vi "Main.vi"() -> ()   [LabVIEW 2019]
doc: "This template is for the Queued Message Handler design pattern.\n\nThe Event Handling Loop generates messages based on user interface actions.\n\nThe Message Handling Loop processes messages generated by the Event Handling Loop, or by other messages. The messages are string values, so new messages can be added easily to the Message Cases case structure in the Message Handling Loop. Each message cluster can also provide an optional value for Message Data, which is a variant that can be converted to whatever message-specific data is required."
uses:
  controls/UI Data.ctl
  support/Message Queue/Enqueue Message (Single).vi
  <vilib>/Utility/error.llb/Error Cluster From Error Code.vi
  <vilib>/ErrorRing/Error Ring.xnode
  support/Message Queue/Message Queue.lvlib
  support/User Event - Stop/User Events.lvlib
panel:
  out "Volts":dbl(knob) scale=0.0..10.0
  out "Display <Replace Me>":string
  in  "Do Something Else <Replace Me>":bool
  in  "Do Something <Replace Me>":bool
  in  "Exit":bool
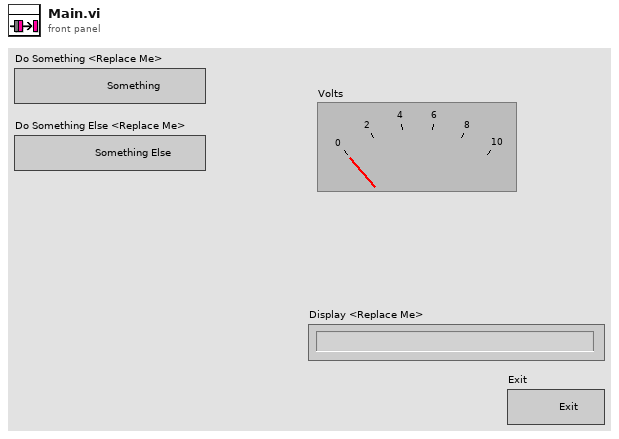
[diagram p1: front panel]
types:
  T1 = typedef "UI Data.ctl" = cluster{"Boolean <Replace Me>":bool, "String <Replace Me>":string, "Numeric <Replace Me>":dbl, "Do Something Ref":refnum<vi>, "Do Something Else Ref":refnum<vi>, "Data Display Ref":refnum<vi>, "Exit Button Ref":refnum<vi>}
  T2 = typedef "User Events.lvlib/User Events Typedef.ctl" = cluster{"Stop Event Interno":refnum<user-event>, "Volts":refnum<user-event>, "QMH Stop":refnum<user-event>, "Stop Event Externo":refnum<user-event>}
  T3 = typedef "Message Queue.lvlib/All Message Queues.ctl" = cluster{"UI":refnum<queue>}
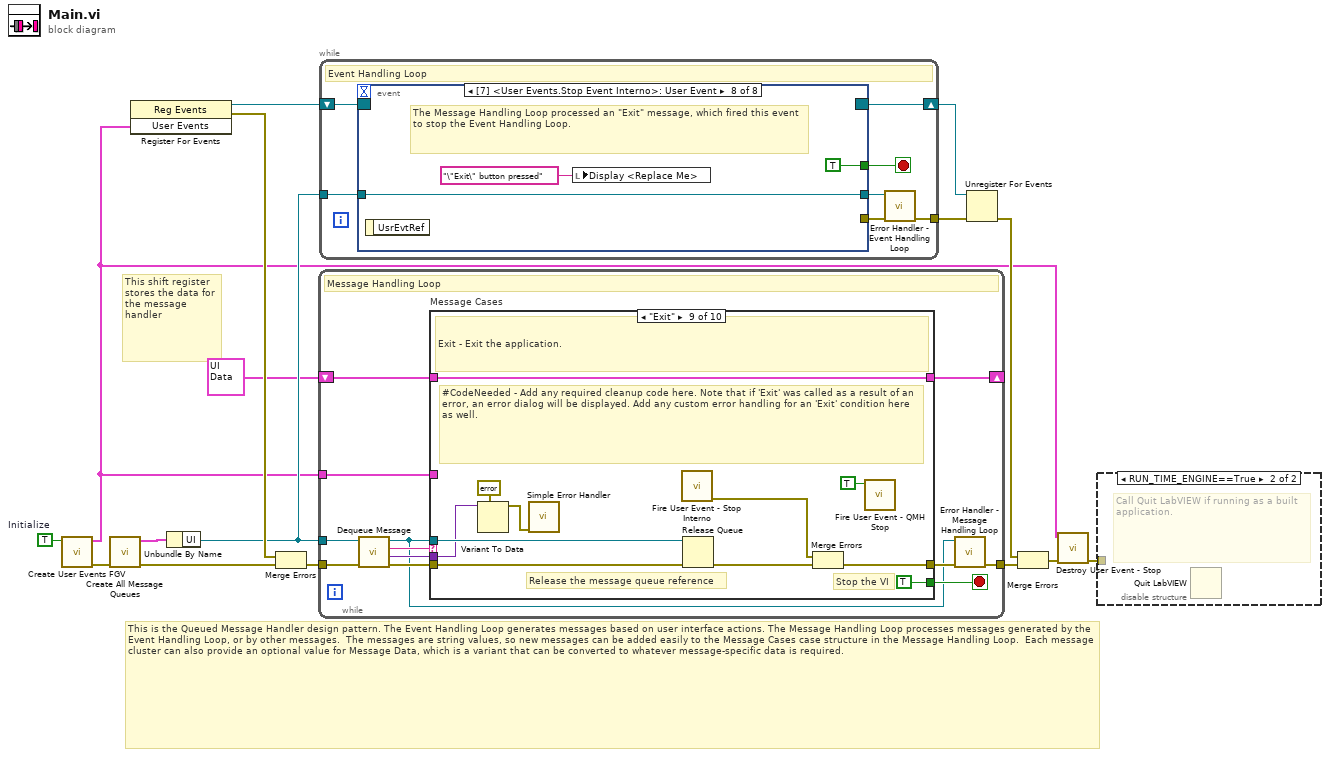
[diagram p0: block diagram]
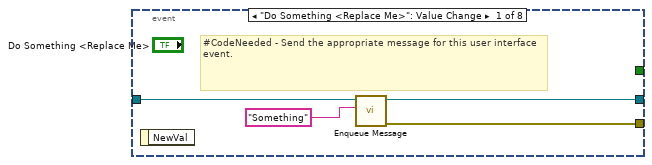
[diagram p3: hidden frame]
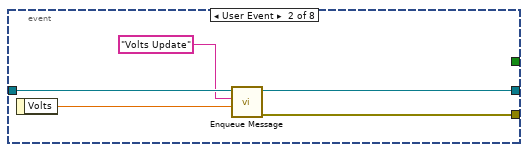
[diagram p4: hidden frame]
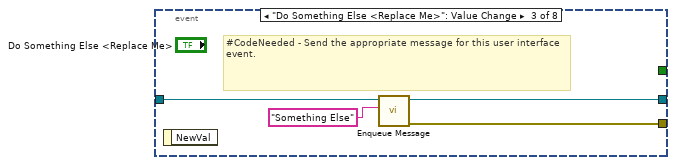
[diagram p5: hidden frame]
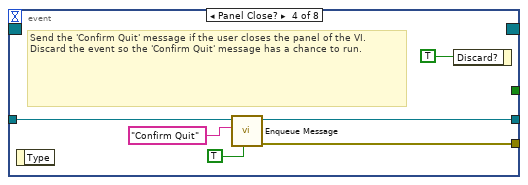
[diagram p6: hidden frame]
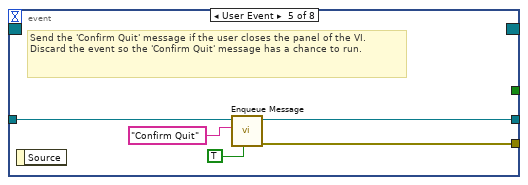
[diagram p7: hidden frame]
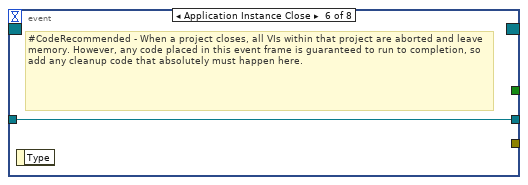
[diagram p8: hidden frame]
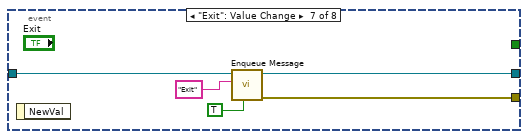
[diagram p9: hidden frame]
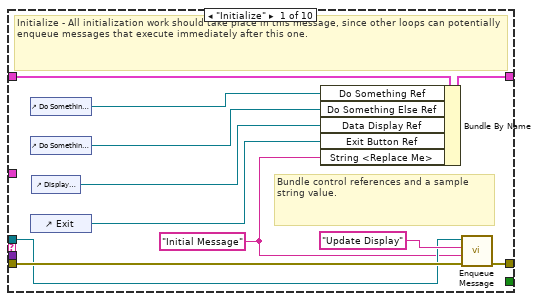
[diagram p10: hidden frame]
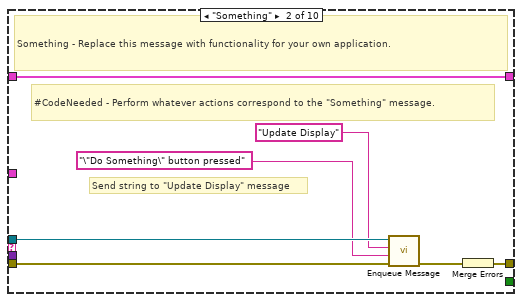
[diagram p11: hidden frame]
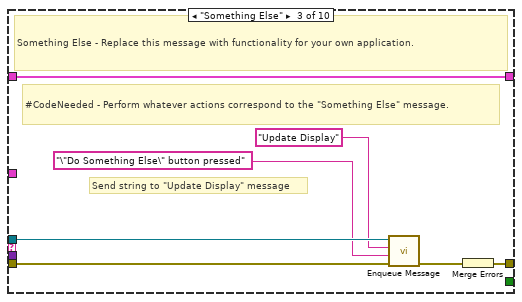
[diagram p12: hidden frame]
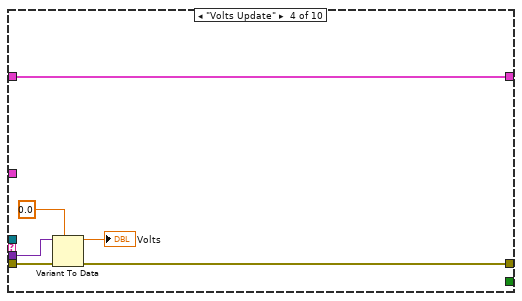
[diagram p13: hidden frame]
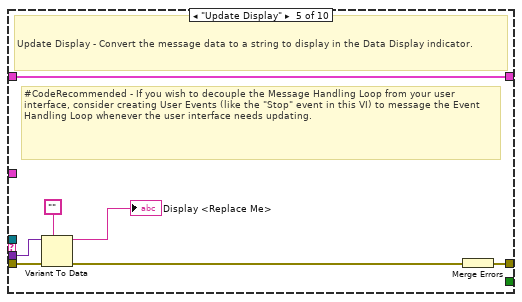
[diagram p14: hidden frame]
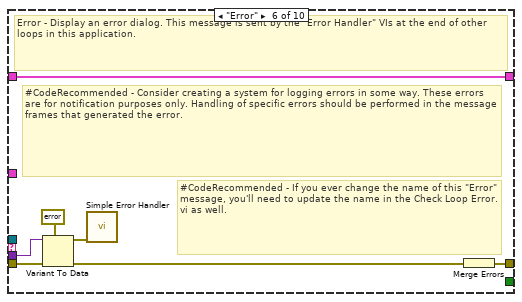
[diagram p15: hidden frame]
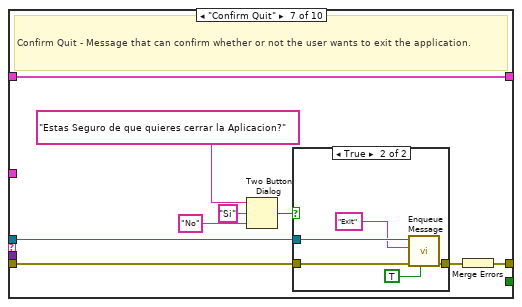
[diagram p16: hidden frame]
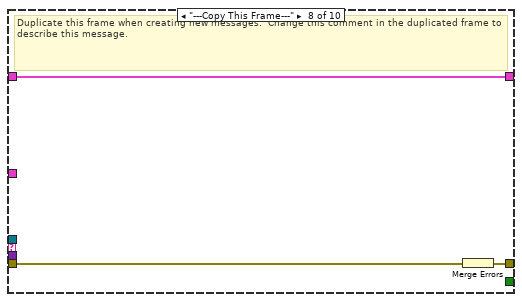
[diagram p18: hidden frame]
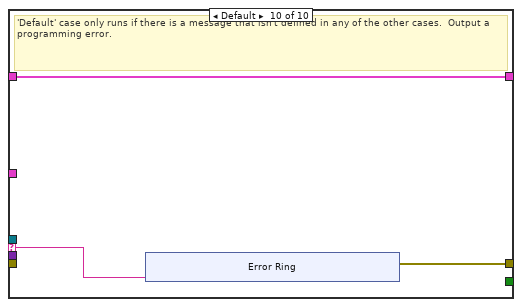
[diagram p19: hidden frame]
diagram:
  w1 = TRUE  # Initialize
  # "This is the Queued Message Handler design pattern. The Event Handling Loop generates messages based on user interface actions. The Message Handling Loop processes messages generated by the Event Handling Loop, or by other messages.  The messages are string values, so new messages can be added easily to the Message Cases case structure in the Message Handling Loop.  Each message cluster can also provide an optional value for Message Data, which is a variant that can be converted to whatever message-specific data is required."
  # "This shift register stores the data for the message handler"
  n1 = call "Create User Events FGV.vi"("Initialize"=w1) -> ("error out"=w14:errorcluster, "User Events"=w2:T2)  [unwired: 9 in]
  n2 = call "Create All Message Queues.vi"("error in (no error)"=w14) -> ("error out"=w16:errorcluster, "Message Queues out"=w7:T3)  [unwired: 9 in]
  n3 = register-events(w2) -> (reference out=w3:refnum<event-registration>, error out=w8:errorcluster)  [unwired: 2 in]
  n4 = Unbundle By Name(w7) -> ("UI"=w6:refnum<queue>)
  n5 = Merge Errors(w8, w16) -> (w9:errorcluster)
  n6 = while {
    tunnel: w6 -> [w18]
    shift-right: [w23] -> _
    shift-left: T1 {"Boolean <Replace Me>"=FALSE, "String <Replace Me>"="", "Numeric <Replace Me>"=0.0, "Do Something Ref"=refnum, "Do Something Else Ref"=refnum, "Data Display Ref"=refnum, "Exit Button Ref"=refnum} ("Data Cluster") -> [w24]
    tunnel: w2 -> [w21]
    tunnel: w9 -> [w28]
    tunnel: [w26] -> w15
    stop <- w22 stop-if-true
    # "Message Handling Loop"
    n7 = call "Dequeue Message.vi"("error in (no error)"=w28, "Message Queue"=w18) -> ("error out"=w27:errorcluster, "Message Data"=w19:variant, "Message"=w20:string, "dup Message Queue"=w17:refnum<queue>)  [unwired: 6 in]
    n8 = case "Message Cases" shown="\"Exit\"" w20 {
      selector: w20 -> [_ _ _ _ _ _ _ _ _ w103]
      tunnel: w17 -> [w30 w42 w49 _ _ _ w78 _ w96 _]
      tunnel: w27 -> [w38 w45 w52 w59 w65 w73 w82 w91 w99 _]
      tunnel: [w39 w46 w53 w58 w66 w69 w81 w90 w101 w105] -> w25
      tunnel: w24 -> [w37 w43 w50 w57 w63 w68 w79 w89 w95 w104]
      tunnel: [w36 w43 w50 w57 w63 w68 w79 w89 w95 w104] -> w23
      tunnel: [_ _ _ _ _ _ _ _ TRUE _] -> w22
      tunnel: w19 -> [_ _ _ w56 w62 w67 _ _ w93 _]
      tunnel: w21 -> [_ _ _ _ _ _ _ _ _ _]
      frame "Initialize" {
        w29 = "Initial Message" ("Initial Message")
        # "Bundle control references and a sample string value."
        # "Initialize - All initialization work should take place in this message, since other loops can potentially enqueue messages that execute immediately after this one."
        n9 = control-ref of="Do Something <Replace Me>"() -> (w35:refnum<vi>)
        n10 = control-ref of="Do Something Else <Replace Me>"() -> (w34:refnum<vi>)
        n11 = control-ref of="Exit"() -> (w32:refnum<vi>)
        n12 = control-ref of="Display <Replace Me>"() -> (w33:refnum<vi>)
        n13 = Bundle By Name(cluster=w37, "Do Something Ref"=w35, "Do Something Else Ref"=w34, "Data Display Ref"=w33, "Exit Button Ref"=w32, "String <Replace Me>"=w29) -> (w36:T1)
        n14 = call-poly "Enqueue Message.vi"("error in (no error)"=w38, "Message Data"=w29, "Message"="Update Display", "Message Queue"=w30) -> ("error out"=w39:errorcluster)  [unwired: 6 in, 1 out]
      }
      frame "Something" {
        # "Send string to \"Update Display\" message"
        # "#CodeNeeded - Perform whatever actions correspond to the \"Something\" message."
        # "Something - Replace this message with functionality for your own application."
        n15 = call-poly "Enqueue Message.vi"("error in (no error)"=w45, "Message Data"="\"Do Something\" button pressed" ("\"Do Something\" button pressed"), "Message"="Update Display", "Message Queue"=w42) -> ("error out"=w44:errorcluster)  [unwired: 6 in, 1 out]
        n16 = Merge Errors(w44) -> (w46:errorcluster)
      }
      frame "Something Else" {
        # "Send string to \"Update Display\" message"
        # "#CodeNeeded - Perform whatever actions correspond to the \"Something Else\" message."
        # "Something Else - Replace this message with functionality for your own application."
        n17 = call-poly "Enqueue Message.vi"("error in (no error)"=w52, "Message Data"="\"Do Something Else\" button pressed" ("\"Do Something Else\" button pressed"), "Message"="Update Display", "Message Queue"=w49) -> ("error out"=w51:errorcluster)  [unwired: 6 in, 1 out]
        n18 = Merge Errors(w51) -> (w53:errorcluster)
      }
      frame "Volts Update" {
        n19 = Variant To Data(error in=w59, type=0.0, Variant=w56) -> (data=→"Volts":dbl, error out=w58:errorcluster)
      }
      frame "Update Display" {
        # "#CodeRecommended - If you wish to decouple the Message Handling Loop from your user interface, consider creating User Events (like the \"Stop\" event in this VI) to message the Event Handling Loop whenever the user interface needs updating."
        # "Update Display - Convert the message data to a string to display in the Data Display indicator."
        n20 = Variant To Data(error in=w65, type="", Variant=w62) -> (data=→"Display <Replace Me>":string, error out=w64:errorcluster)
        n21 = Merge Errors(w64) -> (w66:errorcluster)
      }
      frame "Error" {
        # "#CodeRecommended - If you ever change the name of this \"Error\" message, you'll need to update the name in the Check Loop Error.vi as well."
        # "#CodeRecommended - Consider creating a system for logging errors in some way. These errors are for notification purposes only. Handling of specific errors should be performed in the message frames that generated the error."
        # "Error - Display an error dialog. This message is sent by the \"Error Handler\" VIs at the end of other loops in this application."
        n22 = Variant To Data(error in=w73, type=errorcluster {"status"=FALSE, "code"=0, "source"=""} ("error constant"), Variant=w67) -> (data=w71:errorcluster, error out=w70:errorcluster)
        n23 = call <vilib>:"Simple Error Handler.vi"("error in (no error)"=w71) -> ()  [unwired: 4 in, 5 out]
        n24 = Merge Errors(w70) -> (w69:errorcluster)
      }
      frame "Confirm Quit" {
        # "Confirm Quit - Message that can confirm whether or not the user wants to exit the application."
        n25 = Two Button Dialog(message="Estas Seguro de que quieres cerrar la Aplicacion?", 1:"No" ("T button name (\"OK\")"), 2:"Si" ("T button name (\"OK\")")) -> (T button?=w77:bool)
        n26 = case shown="True" w77 {
          tunnel: w82 -> [w83 w88]
          tunnel: [w83 w87] -> w80
          tunnel: w78 -> [_ w86]
          frame False {
          }
          frame True {
            n27 = call-poly "Enqueue Message.vi"("Priority Message? (F)"=TRUE, "error in (no error)"=w88, "Message"="Exit", "Message Queue"=w86) -> ("error out"=w87:errorcluster)  [unwired: 6 in, 1 out]
          }
        }
        n28 = Merge Errors(w80) -> (w81:errorcluster)
      }
      frame "---Copy This Frame---" {
        # "Duplicate this frame when creating new messages.  Change this comment in the duplicated frame to describe this message."
        n29 = Merge Errors(w91) -> (w90:errorcluster)
      }
      frame "Exit" {
        # "Stop the VI"
        # "Release the message queue reference"
        # "#CodeNeeded - Add any required cleanup code here. Note that if 'Exit' was called as a result of an error, an error dialog will be displayed. Add any custom error handling for an 'Exit' condition here as well."
        # "Exit - Exit the application."
        n30 = Variant To Data(type=errorcluster {"status"=FALSE, "code"=0, "source"=""} ("error constant"), Variant=w93) -> (data=w97:errorcluster)  [unwired: 1 in, 1 out]
        n31 = call <vilib>:"Simple Error Handler.vi"("error in (no error)"=w97) -> ()  [unwired: 4 in, 5 out]
        n32 = call "Fire User Event - Stop Interno.vi"() -> ("error out"=w100:errorcluster)  [unwired: 11 in]
        n33 = Release Queue(queue=w96, error in (no error)=w99) -> (error out=w102:errorcluster)  [unwired: 1 in, 2 out]
        n34 = Merge Errors(w100, w102) -> (w101:errorcluster)
        n35 = call "Fire User Event - QMH Stop.vi"("QMH Stop"=TRUE) -> ()  [unwired: 10 in, 1 out]
      }
      frame Default {
        # "'Default' case only runs if there is a message that isn't defined in any of the other cases.  Output a programming error."
        n36 = xnode "Error Ring"("parameter 0"=w103) -> ("error out"=w105:errorcluster)
      }
    }
    n37 = call "Error Handler - Message Handling Loop.vi"("error in (no error)"=w25, "Message Queue"=w17) -> ("dup error in"=w26:errorcluster)  [unwired: 8 in, 1 out]
  }
  n38 = while {
    tunnel: w6 -> [w117]
    shift-right: [w115] -> w5
    shift-left: w3 -> [w116]
    tunnel: [w118] -> w10
    stop <- w114 stop-if-true
    # "Event Handling Loop"
    n39 = event shown="[7] <User Events.Stop Event Interno>: User Event" {
      selector: w116 -> [_ _ _ _ _ _ _ _]
      dyn-events: [_ _ _ _ _ _ _ _] -> w115
      timeout: _ -> [_ _ _ _ _ _ _ _]
      tunnel: [_ _ _ _ _ _ _ TRUE ("Discard?")] -> w114
      tunnel: w117 -> [w122 w127 w131 w136 w142 w144 w148 w152]
      tunnel: [w123 w128 w132 w138 w143 _ w149 _] -> w119
      tunnel: [w121 w126 w130 w135 w141 w144 w147 w152] -> w113
      event "Do Something <Replace Me>": Value Change {
        # "#CodeNeeded - Send the appropriate message for this user interface event."
        n40 = event-data() -> ()  [unwired: 1 in, 1 out]
        n41 = call-poly "Enqueue Message.vi"("Message"="Something", "Message Queue"=w122) -> ("error out"=w123:errorcluster, "dup Message Queue"=w121:refnum<queue>)  [unwired: 8 in]
      }
      event User Event {
        n42 = event-data() -> ("Volts"=w124:dbl)  [unwired: 1 in]
        n43 = call-poly "Enqueue Message.vi"("Message Data"=w124, "Message"="Volts Update", "Message Queue"=w127) -> ("error out"=w128:errorcluster, "dup Message Queue"=w126:refnum<queue>)  [unwired: 7 in]
      }
      event "Do Something Else <Replace Me>": Value Change {
        # "#CodeNeeded - Send the appropriate message for this user interface event."
        n44 = event-data() -> ()  [unwired: 1 in, 1 out]
        n45 = call-poly "Enqueue Message.vi"("Message"="Something Else", "Message Queue"=w131) -> ("error out"=w132:errorcluster, "dup Message Queue"=w130:refnum<queue>)  [unwired: 8 in]
      }
      event Panel Close? {
        # "Send the 'Confirm Quit' message if the user closes the panel of the VI. Discard the event so the 'Confirm Quit' message has a chance to run."
        n46 = event-data() -> ()  [unwired: 1 in, 1 out]
        n47 = call-poly "Enqueue Message.vi"("Priority Message? (F)"=TRUE, "Message"="Confirm Quit", "Message Queue"=w136) -> ("error out"=w138:errorcluster, "dup Message Queue"=w135:refnum<queue>)  [unwired: 7 in]
        n48 = event-data("Discard?"=TRUE) -> ()  [unwired: 1 in, 1 out]
      }
      event User Event {
        # "Send the 'Confirm Quit' message if the user closes the panel of the VI. Discard the event so the 'Confirm Quit' message has a chance to run."
        n49 = event-data() -> ()  [unwired: 1 in, 1 out]
        n50 = call-poly "Enqueue Message.vi"("Priority Message? (F)"=TRUE, "Message"="Confirm Quit", "Message Queue"=w142) -> ("error out"=w143:errorcluster, "dup Message Queue"=w141:refnum<queue>)  [unwired: 7 in]
      }
      event Application Instance Close {
        # "#CodeRecommended - When a project closes, all VIs within that project are aborted and leave memory. However, any code placed in this event frame is guaranteed to run to completion, so add any cleanup code that absolutely must happen here."
        n51 = event-data() -> ()  [unwired: 1 in, 1 out]
      }
      event "Exit": Value Change {
        n52 = event-data() -> ()  [unwired: 1 in, 1 out]
        n53 = call-poly "Enqueue Message.vi"("Priority Message? (F)"=TRUE, "Message"="Exit", "Message Queue"=w148) -> ("error out"=w149:errorcluster, "dup Message Queue"=w147:refnum<queue>)  [unwired: 7 in]
      }
      event User Event {
        # "The Message Handling Loop processed an \"Exit\" message, which fired this event to stop the Event Handling Loop."
        n54 = event-data() -> ()  [unwired: 1 in, 1 out]
        n55 = local write "Display <Replace Me>"("\"Exit\" button pressed" ("VI Stopped")) -> ()
      }
    }
    n56 = call "Error Handler - Event Handling Loop.vi"("error in (no error)"=w119, "Message Queue"=w113) -> ("dup error in"=w118:errorcluster)  [unwired: 8 in, 1 out]
  }
  n57 = Unregister For Events(event registration refnum=w5, error in=w10) -> (error out=w12:errorcluster)
  n58 = Merge Errors(w12, w15) -> (w13:errorcluster)
  n59 = call "Destroy User Event - Stop.vi"("error in"=w13, "User Events"=w2) -> ("error out"=w11:errorcluster)  [unwired: 9 in]
  n60 = disable-structure shown="RUN_TIME_ENGINE==True" {
    disable-tunnel: w11 -> [_ _]
    frame condition #0 (active) {
    }
    frame condition #1 {
      # "Call Quit LabVIEW if running as a built application."
      n61 = Quit LabVIEW() -> ()  [unwired: 1 in]
    }
  }
